vi "Connection Notify.vi"(8 "error in (no error)":errorcluster, 11 "Head_ScopeSim in":refnum<class "Head_ScopeSim.lvclass">) -> (0 "error out":errorcluster, 3 "Head_ScopeSim out":refnum<class "Head_ScopeSim.lvclass">)   [LabVIEW 2019, in "Head_ScopeSim.lvclass"]
uses:
  Head_ScopeSim.lvclass
  C:/Program Files (x86)/National Instruments/LabVIEW 2019/vi.lib/addons/_Workers/Library/Classes/Worker/Worker.lvclass
  Head_ScopeSim.lvclass/Head_ScopeSim.ctl
  Scope Simulator/rqp_Run Scope.ctl
  gRPC Server/gRPC Server/rqp_Msg_ToClient_1.ctl
  Generated_server/RPC Messages/w4lvgrpc_Msg_ToClient_1.ctl
  gRPC Server/gRPC Server/rqp_Msg_ToClient_3.ctl
  Generated_server/RPC Messages/w4lvgrpc_Msg_ToClient_3.ctl
  Generated_server/RPC Messages/w4lvgrpc_State.ctl
  Scope Simulator/Scope Simulator.lvclass
  gRPC Server/gRPC Server/gRPC Server.lvclass
  Generated_server/Generated_server.lvlib
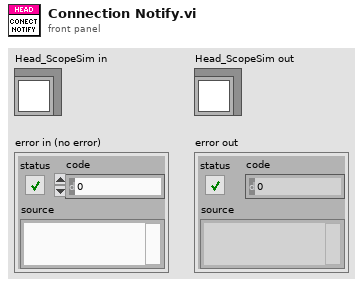
[diagram p1: front panel]
types:
  T1 = typedef "Scope Simulator.lvclass/rqp_Run Scope.ctl" = cluster{"Run Scope ?":bool}
  T2 = typedef "gRPC Server (scope.proto).lvlib/gRPC Server.lvclass/rqp_Msg_ToClient_3.ctl" = cluster{"w4lvgrpc_Msg_ToClient_3":T3}
  T3 = typedef "Generated_server.lvlib/w4lvgrpc_Msg_ToClient_3.ctl" = cluster{"state":T4}
  T4 = typedef "Generated_server.lvlib/w4lvgrpc_State.ctl" = enum32{"STOPPED", "RUNNING", "ERROR"}
  T5 = typedef "gRPC Server (scope.proto).lvlib/gRPC Server.lvclass/rqp_Msg_ToClient_1.ctl" = cluster{"w4lvgrpc_Msg_ToClient_1":T6}
  T6 = typedef "Generated_server.lvlib/w4lvgrpc_Msg_ToClient_1.ctl" = cluster{"device":string, "product_type":string}
  T7 = typedef "Scope Simulator.lvclass/rwr_Get Device Info Reply.ctl" = cluster{"device":string, "product_type":string}
  T8 = typedef "Scope Simulator.lvclass/rwr_Get Scope State Reply.ctl" = cluster{"Scope State":T9}
  T9 = typedef "Scope Simulator.lvclass/rsp_Scope Status.ctl" = enum32{"STOPPED", "RUNNING", "ERROR"}
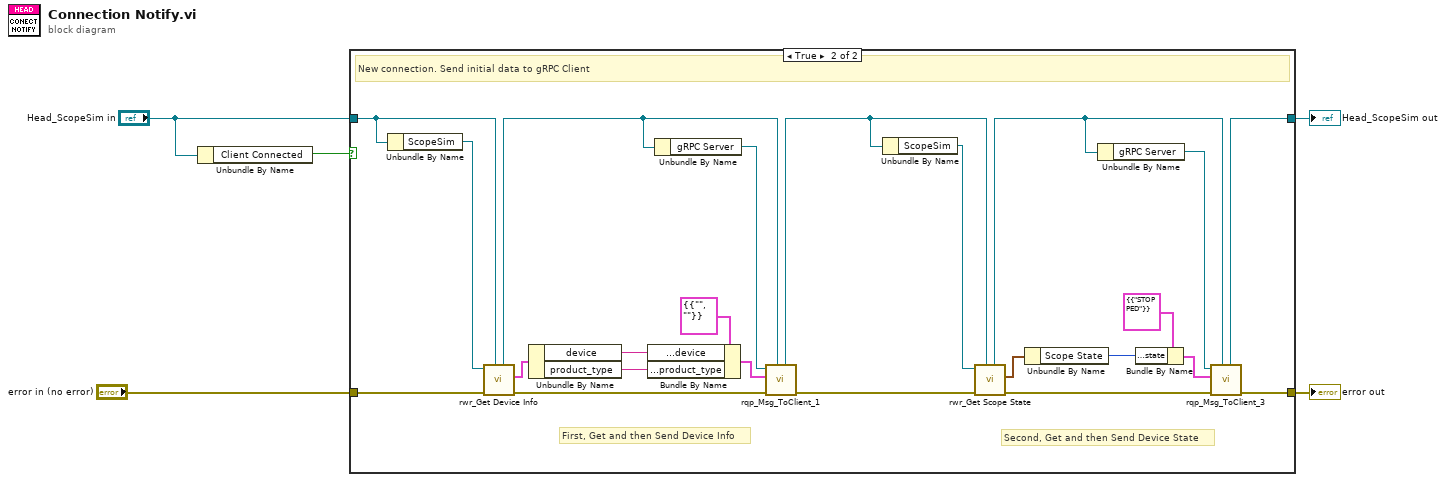
[diagram p0: block diagram]
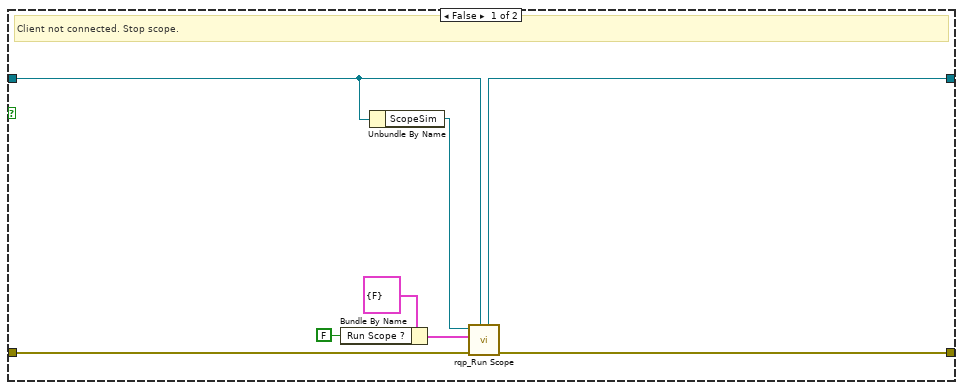
[diagram p2: hidden frame]
diagram:
  n1 = Unbundle By Name("Head_ScopeSim in") -> ("Client Connected"=w1:bool)
  n2 = case shown="True" w1 {
    tunnel: "Head_ScopeSim in" -> [w10 w29]
    tunnel: [w9 w23] -> w3
    tunnel: "error in (no error)" -> [w8 w33]
    tunnel: [w6 w24] -> w5
    frame False {
      # "Client not connected. Stop scope."
      n3 = Bundle By Name(cluster=T1 {"Run Scope ?"=FALSE} ("Data in"), "Run Scope ?"=FALSE) -> (w11:T1)
      n4 = Unbundle By Name(w10) -> ("ScopeSim"=w13:refnum<class "Scope Simulator.lvclass">)
      n5 = call "rqp_Run Scope.vi"("Caller in"=w10, "error in"=w8, "Data in"=w11, "Scope Simulator in"=w13) -> ("error out"=w6:errorcluster, "dup Caller out"=w9:refnum<class "Head_ScopeSim.lvclass">)  [unwired: 5 in, 1 out]
    }
    frame True {
      # "Second, Get and then Send Device State"
      # "First, Get and then Send Device Info"
      # "New connection. Send initial data to gRPC Client"
      n6 = Unbundle By Name(w29) -> ("ScopeSim"=w28:refnum<class "Scope Simulator.lvclass">)
      n7 = call "rwr_Get Device Info.vi"("Caller in"=w29, "error in"=w33, "Scope Simulator in"=w28) -> ("error out"=w31:errorcluster, "Reply Data out"=w27:T7, "dup Caller out"=w30:refnum<class "Head_ScopeSim.lvclass">)  [unwired: 5 in, 1 out]
      n8 = Unbundle By Name(w27) -> ("device"=w26:string, "product_type"=w25:string)
      n9 = Bundle By Name(cluster=T5 {"w4lvgrpc_Msg_ToClient_1"={"device"="", "product_type"=""}} ("Data in"), "w4lvgrpc_Msg_ToClient_1.device"=w26, "w4lvgrpc_Msg_ToClient_1.product_type"=w25) -> (w35:T5)
      n10 = Unbundle By Name(w30) -> ("gRPC Server"=w36:refnum<class "gRPC Server.lvclass">)
      n11 = call "rqp_Msg_ToClient_1.vi"("Caller in"=w30, "error in"=w31, "Data in"=w35, "gRPC Server in"=w36) -> ("error out"=w32:errorcluster, "dup Caller out"=w17:refnum<class "Head_ScopeSim.lvclass">)  [unwired: 5 in, 1 out]
      n12 = Unbundle By Name(w17) -> ("ScopeSim"=w16:refnum<class "Scope Simulator.lvclass">)
      n13 = call "rwr_Get Scope State.vi"("Caller in"=w17, "error in"=w32, "Scope Simulator in"=w16) -> ("error out"=w19:errorcluster, "Reply Data out"=w15:T8, "dup Caller out"=w18:refnum<class "Head_ScopeSim.lvclass">)  [unwired: 5 in, 1 out]
      n14 = Unbundle By Name(w15) -> ("Scope State"=w14:T9)
      n15 = Unbundle By Name(w18) -> ("gRPC Server"=w22:refnum<class "gRPC Server.lvclass">)
      n16 = Bundle By Name(cluster=T2 {"w4lvgrpc_Msg_ToClient_3"={"state"=enum."STOPPED"}} ("Data in"), "w4lvgrpc_Msg_ToClient_3.state"=w14) -> (w20:T2)
      n17 = call "rqp_Msg_ToClient_3.vi"("Caller in"=w18, "error in"=w19, "Data in"=w20, "gRPC Server in"=w22) -> ("error out"=w24:errorcluster, "dup Caller out"=w23:refnum<class "Head_ScopeSim.lvclass">)  [unwired: 5 in, 1 out]
    }
  }
  "error out" <- w5
  "Head_ScopeSim out" <- w3
